vi "SetPosition.vi"(0 "object in":refnum<class "Fruit.lvclass">, 2 "Coordinates":T1, 5 "error in (no error)":errorcluster) -> (14 "object out":refnum<class "Fruit.lvclass">, 19 "error out":errorcluster)   [LabVIEW 2021, in "Fruit.lvclass"]
uses:
  Fruit.lvclass
  Coordinates.ctl
  Fruit.lvclass/Fruit.ctl
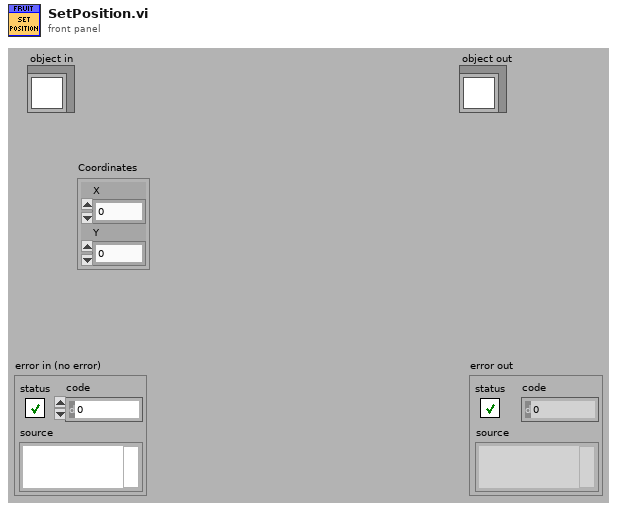
[diagram p1: front panel]
types:
  T1 = typedef "Coordinates.ctl" = cluster{"X":i32, "Y":i32}
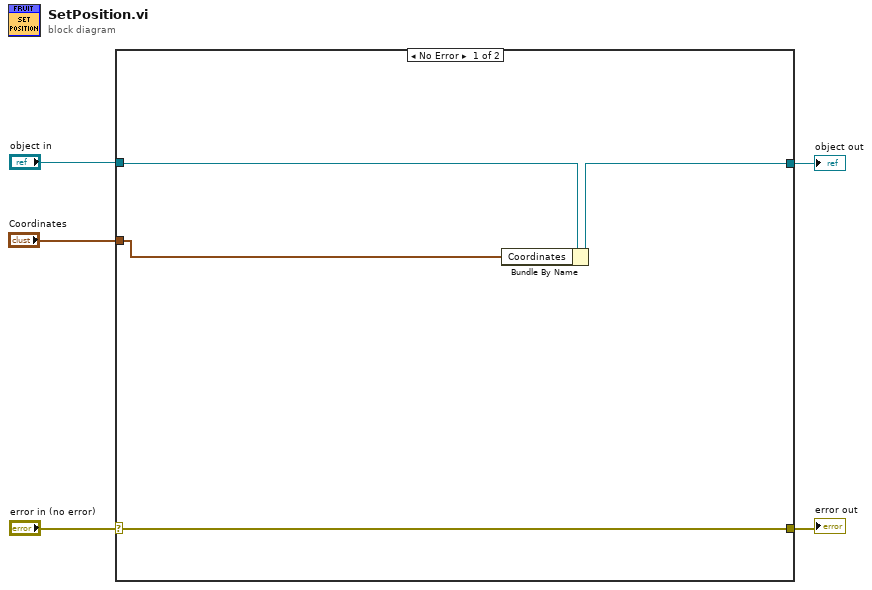
[diagram p0: block diagram]
diagram:
  n1 = case shown="No Error" "error in (no error)" {
    selector: "error in (no error)" -> [w9 w11]
    tunnel: [w9 w11] -> w4
    tunnel: [w7 w10] -> w2
    tunnel: "object in" -> [w8 w10]
    tunnel: "Coordinates" -> [w6 _]
    frame No Error {
      n2 = Bundle By Name(cluster=w8, "Coordinates"=w6) -> (w7:refnum<class "Fruit.lvclass">)
    }
    frame Error {
    }
  }
  "error out" <- w4
  "object out" <- w2
